vi "Enable_Baxter.vi"(0 "error in":errorcluster, 2 "Enable?":bool=TRUE, 3 "node":string) -> (1 "error out":errorcluster)   [LabVIEW 2012]
doc: "This will enable all the motors on Baxter"
uses:
  <userlib>/ROSforLV/ROS/Code/Console/Servers/ServerSubs/TopicDef.ctl
  <userlib>/ROSforLV/ROS/Code/SubVIs/_ROSDirection.ctl
  <userlib>/ROSforLV/ROS/MessageBuilding/std_msgs/subs/boolScalar.vi
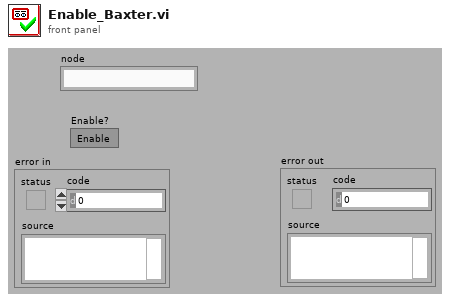
[diagram p1: front panel]
types:
  T1 = typedef "TopicDef.ctl" = cluster{"Topic":string, "Type":string, "Action":T2, "Update (ms)":u16, "write queue":u16}
  T2 = typedef "_ROSDirection.ctl" = enum16{"Node", "Publisher", "Subscriber", "Service Client"}
  T3 = typedef "_ROSControl.ctl" = cluster{"topic port":u16, "Node":string, "topic":string, "type":string, "node port":u16, "error ":errorcluster, "Direction":T2, "APIs":string[], "Update (ms)":u16, "write queue":u16}
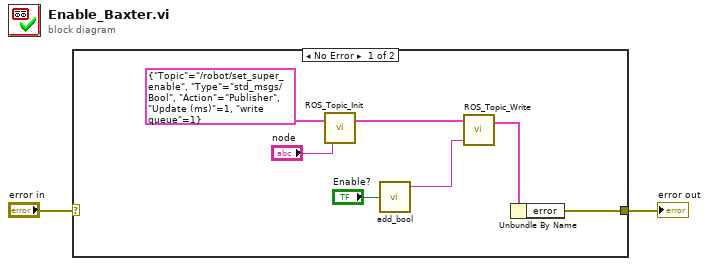
[diagram p0: block diagram]
diagram:
  n1 = case shown="No Error" "error in" {
    selector: "error in" -> [_ w10]
    tunnel: [w7 w10] -> w2
    frame No Error {
      n2 = call <userlib>:"ROS_Topic_Init.vi"("node"="node", "Definitions"=T1 {"Topic"="/robot/set_super_enable", "Type"="std_msgs/Bool", "Action"=enum."Publisher", "Update (ms)"=1, "write queue"=1}) -> ("ROS out"=w9:T3)  [unwired: 1 in]
      n3 = call-poly <userlib>:"add_bool.vi"("Boolean"="Enable?") -> ("msg out"=w5:string)  [unwired: 4 in]
      n4 = call <userlib>:"ROS_Topic_Write.vi"("Msg in"=w5, "ROS in"=w9) -> ("ROS out"=w8:T3)  [unwired: 2 in]
      n5 = Unbundle By Name(w8) -> ("error"=w7:errorcluster)
    }
    frame Error {
    }
  }
  "error out" <- w2
